vi "PH_StatusHandler.set Status GUI Object.vi"(2 "PH Status Ref":refnum<vi>, 3 "Value":T1 items=["no info", "off/false/out", "on/true/in", "Failure", "Alarm", "Status 1", "Status 2", "Status 3"], 4 "Blinking (false)":bool, 5 "error in (no error)":errorcluster, 7 "Tip Strip":string="N/A") -> (19 "error out":errorcluster)   [LabVIEW 2014, in "PH_StatusHandler.lvlib"]
doc: "This VI sets the value of a Status (a strict type def I16 Ring object) if the reference is valid."
uses:
  PH_StatusHandler.Status.ctl
  PH_StatusHandler.GUI element.ctl
  PH_StatusHandler.lvlib
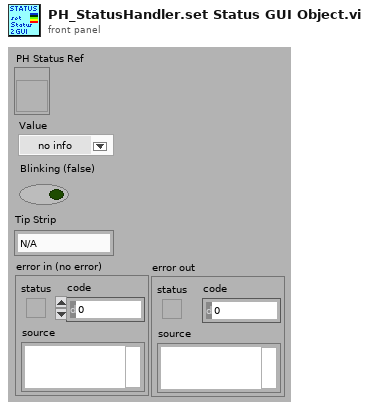
[diagram p1: front panel]
types:
  T1 = typedef "PH_StatusHandler.lvlib/PH_StatusHandler.Status.ctl" = i16
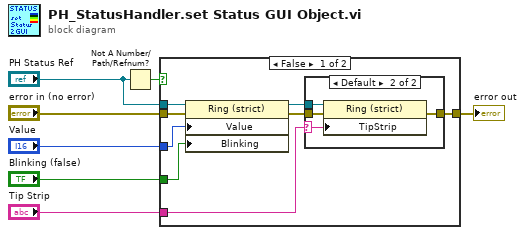
[diagram p0: block diagram]
diagram:
  n1 = Not A Number/Path/Refnum?(number/path/refnum="PH Status Ref") -> (NaN/Path/Refnum?=w4:bool)
  n2 = case shown="False" w4 {
    tunnel: "error in (no error)" -> [w15 w21]
    tunnel: [w11 w21] -> w5
    tunnel: "PH Status Ref" -> [w14 _]
    tunnel: "Value" -> [w8 _]
    tunnel: "Blinking (false)" -> [w13 _]
    tunnel: "Tip Strip" -> [w9 _]
    frame False {
      n3 = property class="Ring (strict)"(reference=w14, error in=w15, "Value"=w8, "Blinking"=w13) -> (reference out=w10:refnum<vi>, error out=w12:errorcluster)
      n4 = case shown="Default" w9 {
        selector: w9 -> [_ w17]
        tunnel: w12 -> [w16 w20]
        tunnel: [w16 w19] -> w11
        tunnel: w10 -> [_ w18]
        frame "", "N/A" {
        }
        frame Default {
          n5 = property class="Ring (strict)"(reference=w18, error in=w20, "TipStrip"=w17) -> (error out=w19:errorcluster)  [unwired: 1 out]
        }
      }
    }
    frame True {
    }
  }
  "error out" <- w5
